vi "Collection Logic.vi"(6 "Valid Path?":bool, 7 "File Path":path, 9 "START/STOP":bool, 11 "Saving Data":bool) -> (0 "Camera Button Disabled?":T1(ring), 1 "Start/Stop Disabled?":T1(ring), 2 "Exit Disabled?":T1(ring), 3 "First or After?":bool, 4 "Warn User":bool)   [LabVIEW 2020, in "SubVIs.lvlib"]
uses:
  SubVIs.lvlib
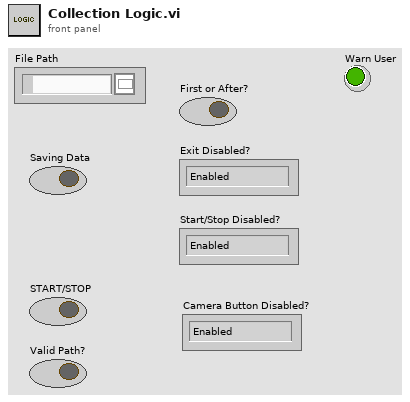
[diagram p1: front panel]
types:
  T1 = enum8{"Enabled", "Disabled", "Disabled and Grayed Out"}
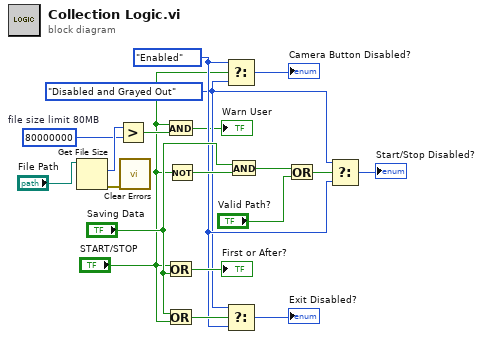
[diagram p0: block diagram]
diagram:
  w6 = i64 80000000  # file size limit 80MB
  w8 = T1."Disabled and Grayed Out" ("t")
  w9 = T1."Enabled" ("Disabled")
  n1 = Get File Size(file="File Path") -> (size (in bytes)=w7:i64, 0:w4:errorcluster)  [unwired: 1 in, 1 out]
  n2 = Greater?(x=w7, y=w6) -> (0:w3:bool)
  n3 = call <vilib>:"Clear Errors.vi"("error in (no error)"=w4) -> ()  [unwired: 5 in, 2 out]
  n4 = And(x="START/STOP", y=w3) -> (x .and. y?=→"Warn User":bool)
  n5 = Or(x="START/STOP", y="Saving Data") -> (x .or. y?=→"First or After?":bool)
  n6 = Or(x="Saving Data", y="START/STOP") -> (x .or. y?=w14:bool)
  n7 = Not(x="START/STOP") -> (.not. x?=w11:bool)
  n8 = Select(t=w9, s="START/STOP", f=w8) -> (s? t:f=→"Camera Button Disabled?":T1)
  n9 = Select(t=w8, s=w14, f=w9) -> (s? t:f=→"Exit Disabled?":T1)
  n10 = And(x="Saving Data", y=w11) -> (x .and. y?=w10:bool)
  n11 = Or(x=w10, y="Valid Path?") -> (x .or. y?=w16:bool)
  n12 = Select(t=w8, s=w16, f=w9) -> (s? t:f=→"Start/Stop Disabled?":T1)
